vi "GetData_subVI.vi"(9 "word after":string, 10 "word before":string, 11 "body in":string) -> (3 "data out":string)   [LabVIEW 2015]
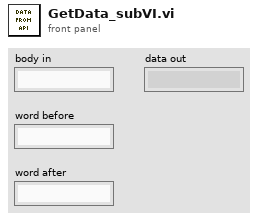
[diagram p1: front panel]
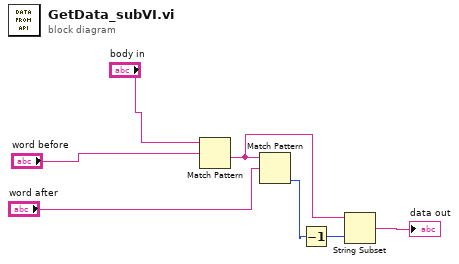
[diagram p0: block diagram]
diagram:
  n1 = Match Pattern(string="body in", regular expression="word before") -> (after substring=w4:string)  [unwired: 1 in, 3 out]
  n2 = Match Pattern(string=w4, regular expression="word after") -> (offset past match=w6:i32)  [unwired: 1 in, 3 out]
  n3 = Decrement(x=w6) -> (x-1=w7:i32)
  n4 = String Subset(string=w4, length (rest)=w7) -> (substring=→"data out":string)  [unwired: 1 in]
